vi "Temperature_Limits.vi"(6 "Temp limits":T1={"Max (25)"=25.0, "Min (0)"=0.0}, 8 "error in (no error)":errorcluster, 10 "TEMP":dbl) -> (0 "error out":errorcluster, 2 "Warning":bool, 3 "Warning Text":string)   [LabVIEW 2014]
doc: "SubVI porównuje temperaturę\nprocesową z zadanymi wartościami granicznymi"
uses:
  inne pliki/Params.ctl
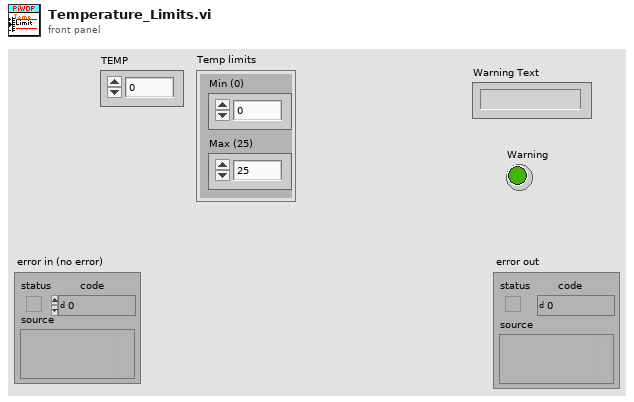
[diagram p1: front panel]
types:
  T1 = typedef "Params.ctl" = cluster{"Max (25)":dbl, "Min (0)":dbl}
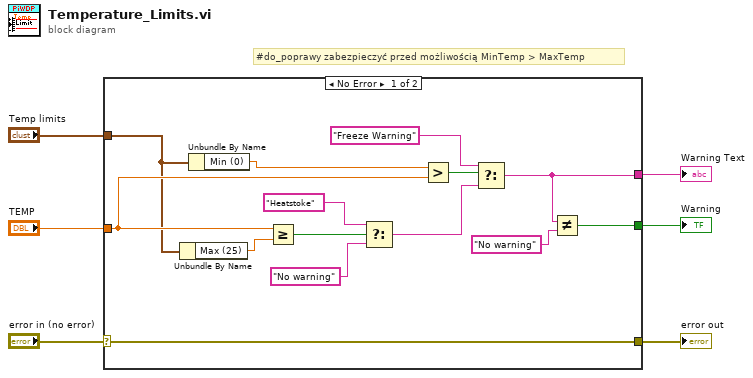
[diagram p0: block diagram]
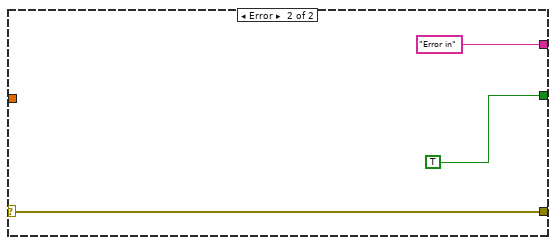
[diagram p2: hidden frame]
diagram:
  # "#do_poprawy zabezpieczyć przed możliwością MinTemp > MaxTemp"
  n1 = case shown="No Error" "error in (no error)" {
    selector: "error in (no error)" -> [w10 w23]
    tunnel: [w10 w23] -> w5
    tunnel: "TEMP" -> [w17 _]
    tunnel: [w13 "Error in"] -> w3
    tunnel: [w11 TRUE] -> w2
    tunnel: "Temp limits" -> [w8 _]
    frame No Error {
      n2 = Unbundle By Name(w8) -> ("Max (25)"=w9:dbl)
      n3 = Unbundle By Name(w8) -> ("Min (0)"=w7:dbl)
      n4 = Greater Or Equal?(x=w17, y=w9) -> (x >= y?=w20:bool)
      n5 = Select(t="Heatstoke", s=w20, f="No warning") -> (s? t:f=w15:string)
      n6 = Greater?(x=w7, y=w17) -> (0:w16:bool)
      n7 = Select(t="Freeze Warning", s=w16, f=w15) -> (s? t:f=w13:string)
      n8 = Not Equal?(x=w13, y="No warning") -> (x != y?=w11:bool)
    }
    frame Error {
    }
  }
  "error out" <- w5
  "Warning Text" <- w3
  "Warning" <- w2
